vi "日期字符串格式至时间格式转换.vi"(10 "格式字符串":string="%d-%d-%d %d-%d-%d", 11 "time":string) -> (3 "time stamp":timestamp format="%<%Y/%m/%d %H:%M:%S>T")   [LabVIEW 2016, in "工况数据上传.lvlib"]
uses:
  <vilib>/Utility/miscctls.llb/LVDateTimeRec.ctl
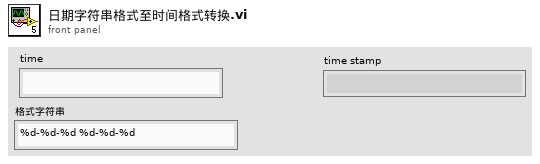
[diagram p1: front panel]
types:
  T1 = typedef "LVDateTimeRec.ctl" = cluster{"fractional second":dbl, "second":i32, "minute":i32, "hour":i32, "day of month":i32, "month":i32, "year":i32, "day of week":i32, "day of year":i32, "DST":i32}
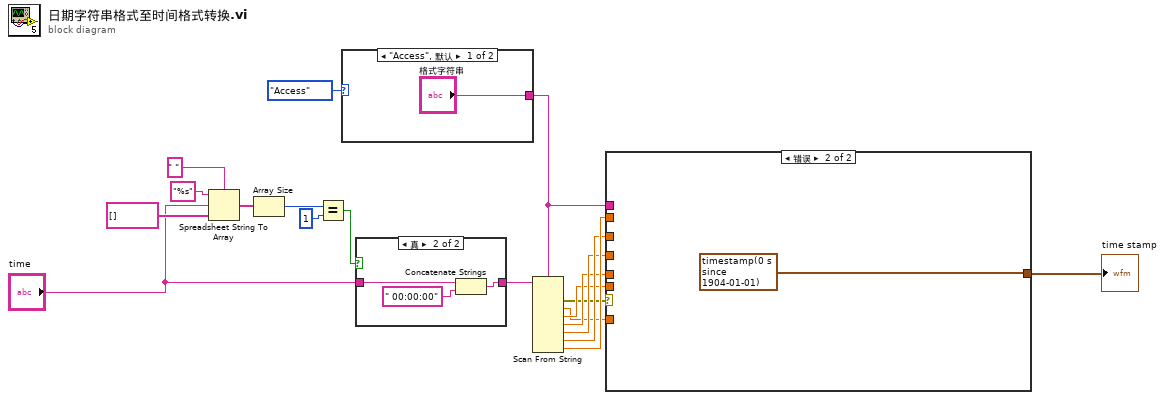
[diagram p0: block diagram]
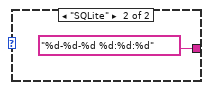
[diagram p2: hidden frame]
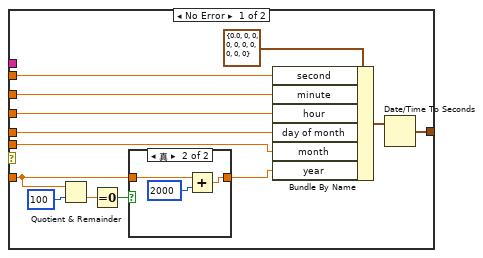
[diagram p4: hidden frame]
diagram:
  n1 = Spreadsheet String To Array(delimiter (Tab)=" " ("分隔符(Tab)"), format string="%s" ("格式字符串"), spreadsheet string="time", array type (2D Dbl)=string[] []) -> (array=w8:string[])
  n2 = Array Size(array=w8) -> (size(s)=w7:i32)
  n3 = Equal?(x=w7, y=1) -> (x = y?=w5:bool)
  n4 = case shown="\"Access\", 默认" enum16{"Access", "SQLite"}."Access" ("数据库类型") {
    tunnel: ["格式字符串" "%d-%d-%d %d:%d:%d" ("格式字符串")] -> w1
    frame "Access", Default {
    }
    frame "SQLite" {
    }
  }
  n5 = case shown="真" w5 {
    tunnel: "time" -> [w22 w24]
    tunnel: [w22 w23] -> w3
    frame False {
    }
    frame True {
      n6 = Concatenate Strings(w24, " 00:00:00" ("字符串")) -> (w23:string)
    }
  }
  n7 = Scan From String(format string=w1, input string=w3) -> (error out=w13:errorcluster, output 1=w14:dbl, output 2=w15:dbl, output 3=w16:dbl, output 4=w17:dbl, output 5=w18:dbl, output 6=w19:dbl)  [unwired: 8 in, 2 out]
  n8 = case shown="错误" w13 {
    tunnel: w19 -> [w37 _]
    tunnel: w18 -> [w36 _]
    tunnel: w17 -> [w35 _]
    tunnel: w16 -> [w34 _]
    tunnel: w15 -> [w33 _]
    tunnel: w14 -> [w29 _]
    tunnel: [w31 timestamp(0 s since 1904-01-01) ("time stamp")] -> w12
    tunnel: w1 -> [_ _]
    frame No Error {
      n9 = Quotient & Remainder(x=w29, y=100) -> (floor(x/y)=w28:dbl)  [unwired: 1 out]
      n10 = Equal To 0?(x=w28) -> (x = 0?=w27:bool)
      n11 = case shown="真" w27 {
        tunnel: w29 -> [w39 w42]
        tunnel: [w39 w40] -> w26
        frame False {
        }
        frame True {
          n12 = Add(x=w42, y=2000) -> (x+y=w40:dbl)
        }
      }
      n13 = Bundle By Name(cluster=T1 {"fractional second"=0.0, "second"=0, "minute"=0, "hour"=0, "day of month"=0, "month"=0, "year"=0, "day of week"=0, "day of year"=0, "DST"=0} ("日期时间记录"), "second"=w37, "minute"=w36, "hour"=w35, "day of month"=w34, "month"=w33, "year"=w26) -> (w38:T1)
      n14 = Date/Time To Seconds(2:w38) -> (0:w31:timestamp)  [unwired: 1 in]
    }
    frame Error {
    }
  }
  "time stamp" <- w12
